vi "Set Counter Configuration.vi"(8 "error in":errorcluster, 10 "Max Count":dbl, 11 "Parent Ref":T1=18446744073709551615 format="%.0x") -> (0 "error out":errorcluster, 3 "Parent Ref Out":T1=18446744073709551615 format="%.0x")   [LabVIEW 2015, in "Protection and Rolling Counter Addon System Explorer.lvlib"]
uses:
  <vilib>/NI Veristand/Custom Device API/Custom Device Item Ref.ctl
  Shared/SubVIs/GUID Lookup.vi
  <vilib>/NI Veristand/Custom Device API/Set Item Property (Variant).vi
  Protection and Rolling Counter Addon System Explorer.lvlib
  <vilib>/NI Veristand/Custom Device API/Custom Device API.lvlib
  Shared/Protection and Rolling Counter Addon Shared.lvlib
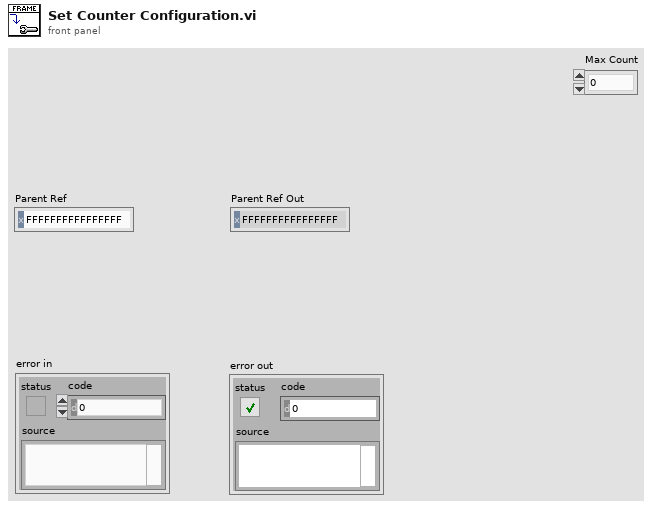
[diagram p1: front panel]
types:
  T1 = typedef "Custom Device API.lvlib/Custom Device Item Ref.ctl" = u64
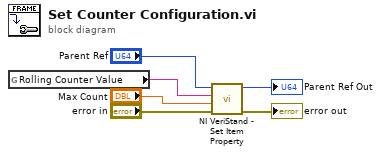
[diagram p0: block diagram]
diagram:
  n1 = global read "GUID Lookup.vi" "Rolling Counter Value"() -> (w2:string)
  n2 = call-poly <vilib>:"NI VeriStand - Set Item Property.vi"("error in (no error)"="error in", "Value"="Max Count", "Property Name"=w2, "Item Ref in"="Parent Ref") -> ("error out"=→"error out":errorcluster, "Item Ref out"=→"Parent Ref Out":T1)  [unwired: 5 in, 1 out]
